vi "Set_Active_Device.vi"(8 "error in (no error)":errorcluster, 9 "Init Fingers":bool, 10 "device":T1) -> (0 "error out":errorcluster)   [LabVIEW 2019, in "Kinova MICO² USB.lvlib"]
uses:
  <vilib>/Utility/error.llb/Error Cluster From Error Code.vi
  <vilib>/ErrorRing/Error Ring.xnode
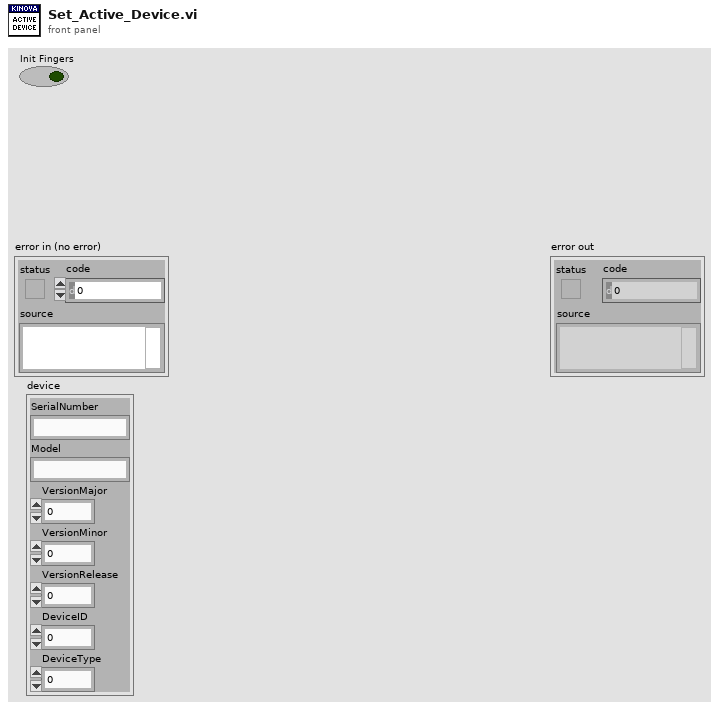
[diagram p1: front panel]
types:
  T1 = cluster{"SerialNumber":string, "Model":string, "VersionMajor":i32, "VersionMinor":i32, "VersionRelease":i32, "DeviceID":i32, "DeviceType":i32}
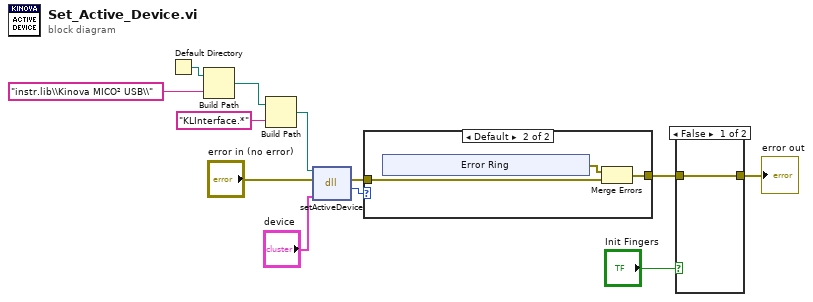
[diagram p0: block diagram]
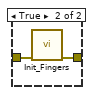
[diagram p2: hidden frame]
diagram:
  n1 = Default Directory() -> (w6:path)
  n2 = Build Path(base path=w6, name or relative path="instr.lib\\Kinova MICO² USB\\") -> (appended path=w4:path)
  n3 = Build Path(base path=w4, name or relative path="KLInterface.*") -> (appended path=w7:path)
  n4 = dll-call lib="C:/Users/mcjssdcc/source/repos/Kinova Labview Interface/Debug/KLInterface.dll" fn="setActiveDevice"(path in=w7, error in="error in (no error)", "device"="device") -> (error out=w10:errorcluster, "return type"=w9:i32)  [unwired: 2 in, 1 out]
  n5 = case shown="Default" w9 {
    tunnel: [w13 w15] -> w3
    tunnel: w10 -> [w13 w14]
    frame 1 {
    }
    frame Default {
      n6 = xnode "Error Ring"() -> ("error out"=w16:errorcluster)
      n7 = Merge Errors(w16, w14) -> (w15:errorcluster)
    }
  }
  n8 = case shown="False" "Init Fingers" {
    tunnel: w3 -> [w22 w24]
    tunnel: [w22 w23] -> w2
    frame False {
    }
    frame True {
      n9 = call "Init_Fingers.vi"("error in (no error)"=w24) -> ("error out"=w23:errorcluster)  [unwired: 10 in]
    }
  }
  "error out" <- w2
